vi "EOL CAN_Send_Two_Part_Message (2).vi"(0 "Write Session in":refnum<k21>, 1 "Rx Arbitration Id":u32=402522244 format="%.0x", 5 "Read Session in":refnum<k21>, 7 "Tx CAN frame 1":T1={"timestamp"=timestamp(0 s since 1904-01-01), "payload"=[2, 39, 3, 85, 85, 85, 85, 85], "identifier"=402391172, "type"=0, "extended?"=TRUE, "echo?"=FALSE} {"payload" format="%x"; "timestamp" format="%<%.7X\n%x>T"; "type" items=["CAN Data"=0, "CAN Remote"=1, "CAN Bus Error"=2, "CAN 2.0 Data"=8, "CAN FD Data"=16, "CAN FD+BRS Data"=24, "J1939 Data"=192, "Delay"=224, "Log Trigger"=225, "Start Trigger"=226]; "identifier" format="%x"}, 9 "Tx CAN frame 2":T1={"timestamp"=timestamp(0 s since 1904-01-01), "payload"=[2, 39, 3, 85, 85, 85, 85, 85], "identifier"=402391172, "type"=0, "extended?"=TRUE, "echo?"=FALSE} {"payload" format="%x"; "timestamp" format="%<%.7X\n%x>T"; "type" items=["CAN Data"=0, "CAN Remote"=1, "CAN Bus Error"=2, "CAN 2.0 Data"=8, "CAN FD Data"=16, "CAN FD+BRS Data"=24, "J1939 Data"=192, "Delay"=224, "Log Trigger"=225, "Start Trigger"=226]; "identifier" format="%x"}, 11 "error in (no error)":errorcluster, 12 "Retries":i32=1, 13 "Msg Wait Time":u32=100) -> (4 "Response Good?":bool, 6 "Rx Data":u8[](array[numeric]), 10 "TxRx Data":string[][](array[string]), 15 "error out":errorcluster)   [LabVIEW 2018]
uses:
  <vilib>/xnet/xnet.llb/XNET Frame CAN.ctl
  <vilib>/xnet/xnet.llb/XNET Frame Type CAN.ctl
  <vilib>/xnet/xnet.llb/XNET Write (Frame CAN).vi
  <vilib>/xnet/xnet.llb/XNET Read (Frame CAN).vi
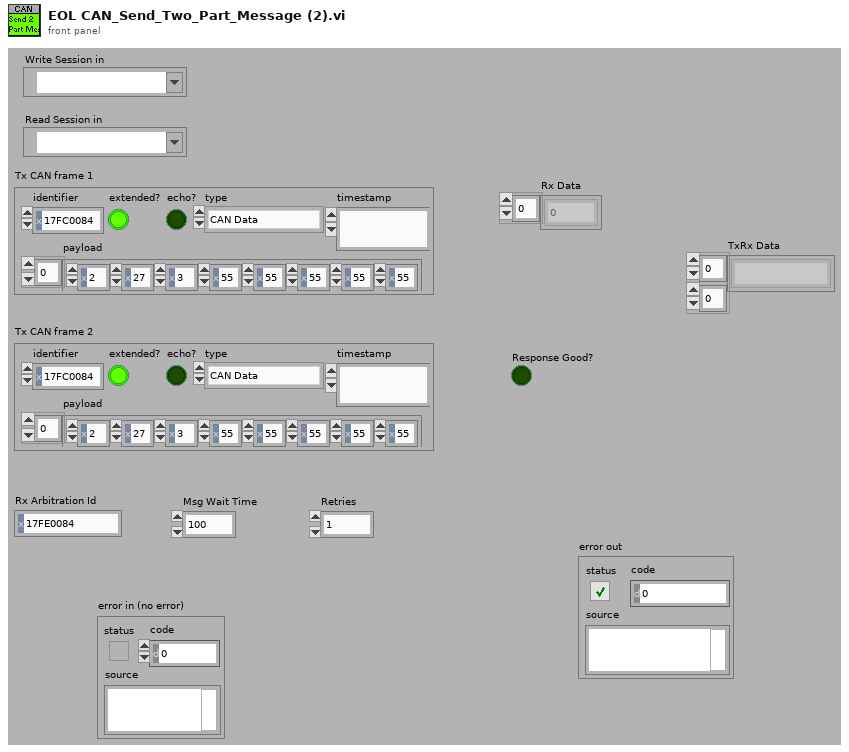
[diagram p1: front panel]
types:
  T1 = typedef "XNET Frame CAN.ctl" = cluster{"timestamp":timestamp, "payload":u8[], "identifier":u32, "type":T2, "extended?":bool, "echo?":bool}
  T2 = typedef "XNET Frame Type CAN.ctl" = u8
  T3 = cluster{"Write Session in":refnum<k21>, "Read Session in":refnum<k21>, "Tx CAN frame 1":T1, "Tx CAN frame 2":T1, "Rx Arbitration Id":u32, "Retry Counter":i32, "Rx Data":u8[], "Response Good?":bool, "TxRx Data":string[][], "Rx Bytes Length":u8, "error in (no error)":errorcluster}
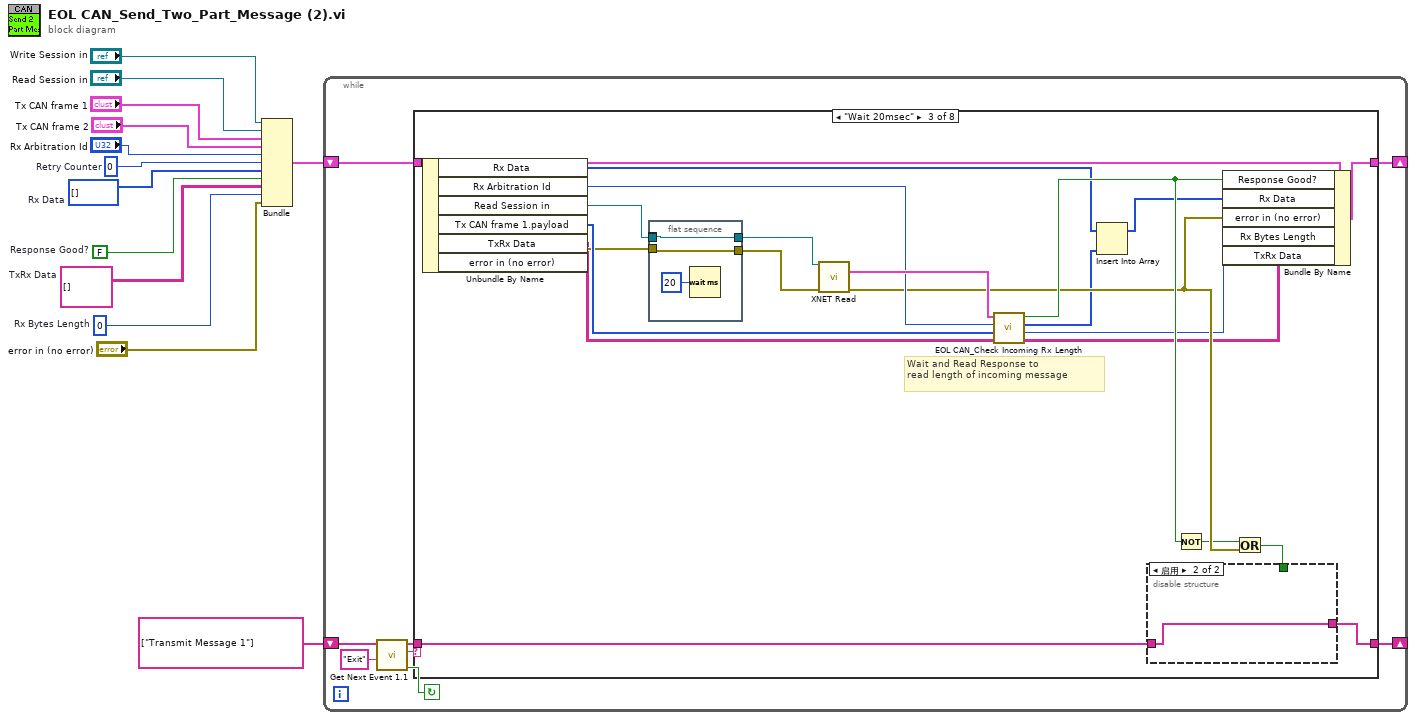
[diagram p0: block diagram]
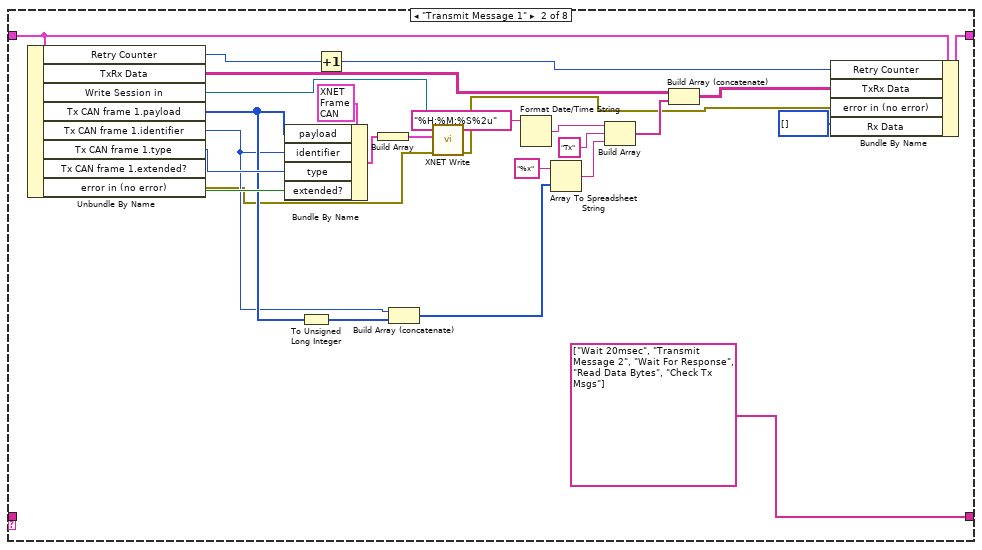
[diagram p3: hidden frame]
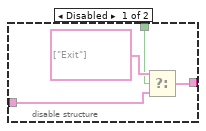
[diagram p4: hidden frame]
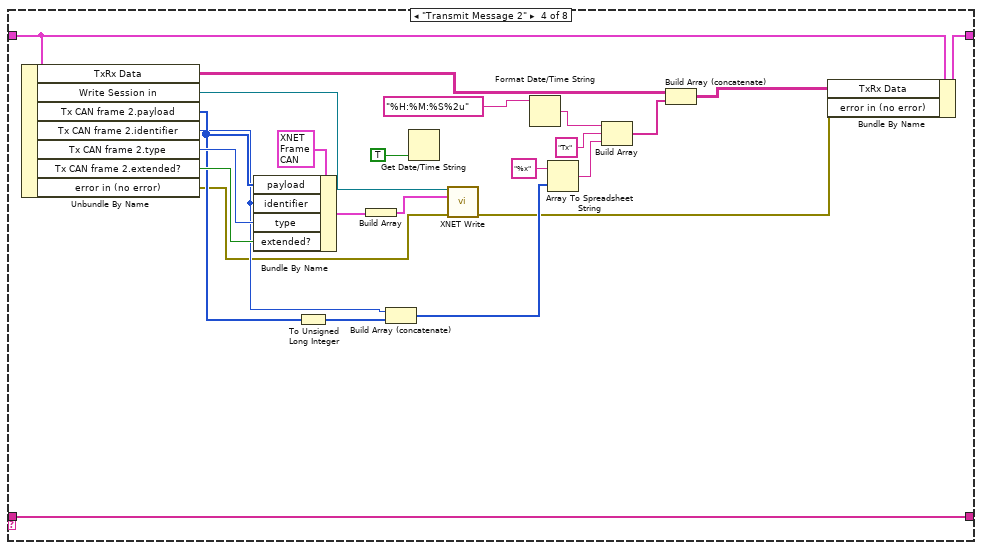
[diagram p5: hidden frame]
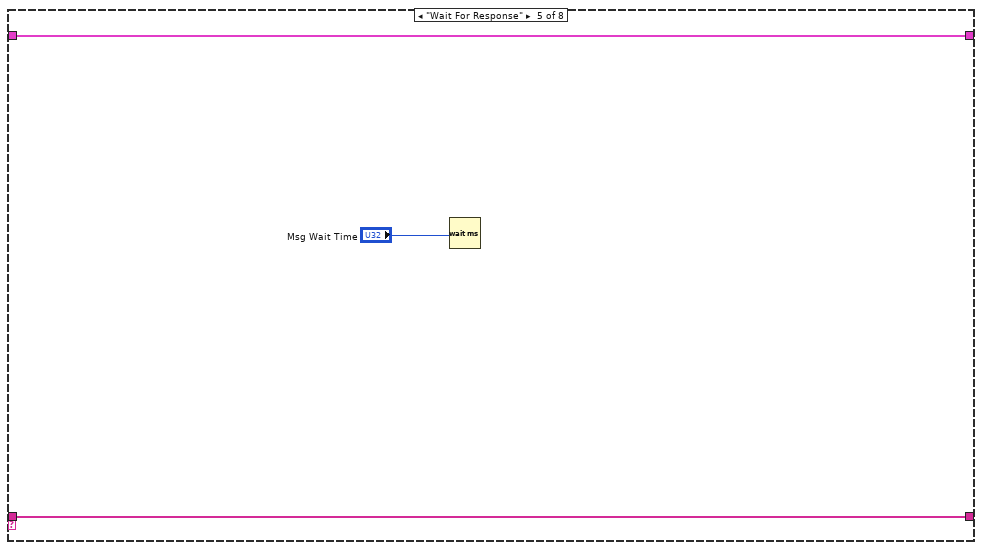
[diagram p6: hidden frame]
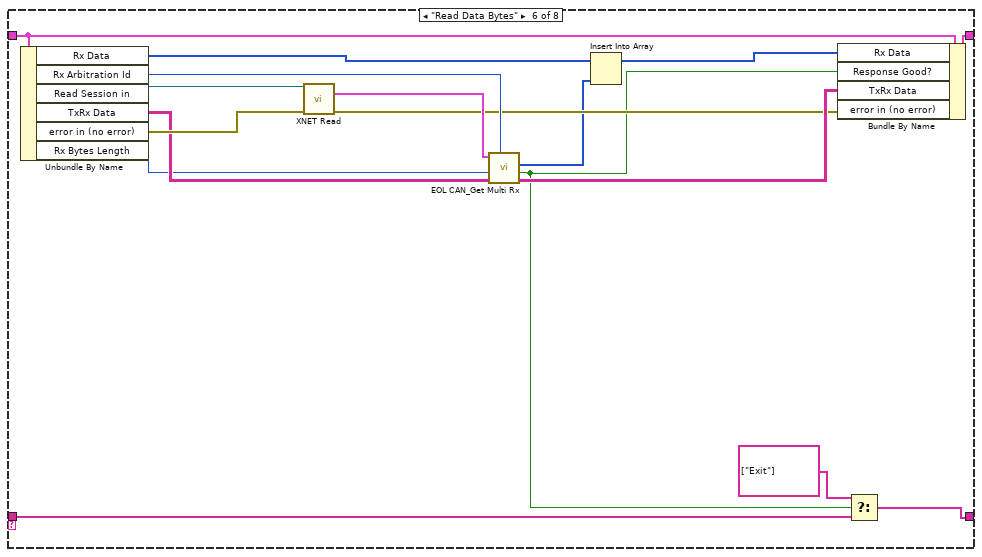
[diagram p7: hidden frame]
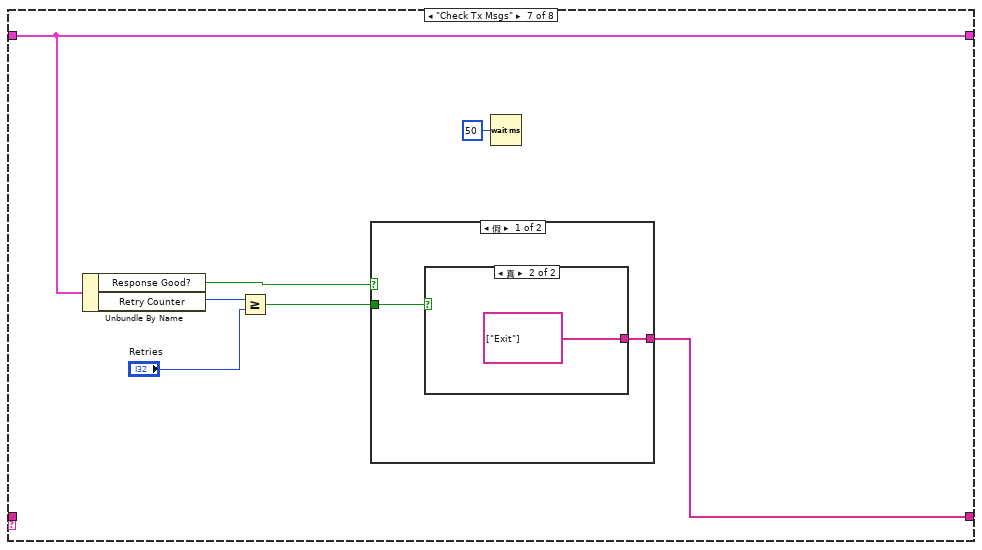
[diagram p8: hidden frame]
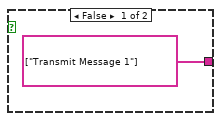
[diagram p9: hidden frame]
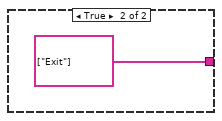
[diagram p10: hidden frame]
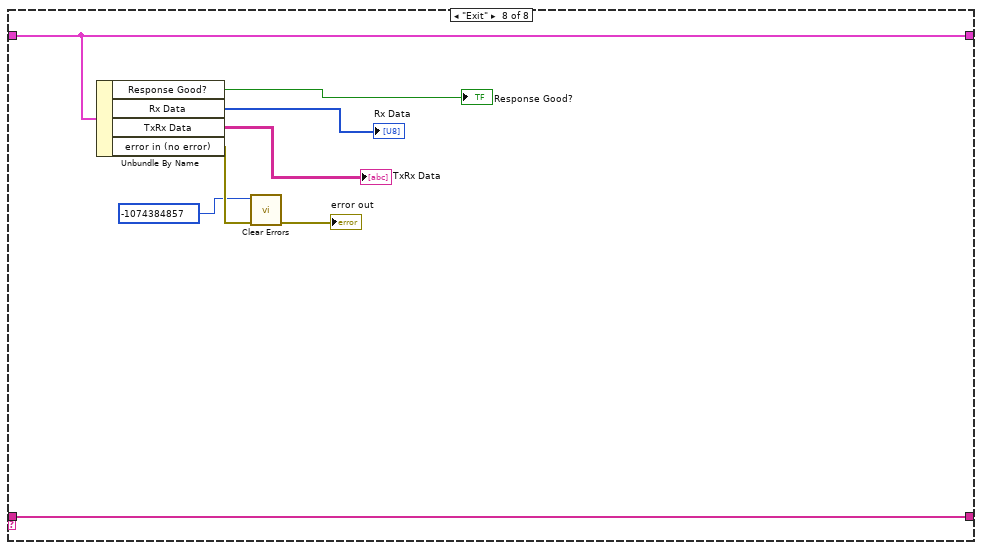
[diagram p11: hidden frame]
diagram:
  w1 = u8[] []  # Rx Data
  w2 = u8 0  # Rx Bytes Length
  w9 = string[][] []  # TxRx Data
  w10 = FALSE  # Response Good?
  w12 = 0  # Retry Counter
  n1 = Bundle("Write Session in"="Write Session in", "Read Session in"="Read Session in", "Tx CAN frame 1"="Tx CAN frame 1", "Tx CAN frame 2"="Tx CAN frame 2", "Rx Arbitration Id"="Rx Arbitration Id", "Retry Counter"=w12, "Rx Data"=w1, "Response Good?"=w10, "TxRx Data"=w9, "Rx Bytes Length"=w2, "error in (no error)"="error in (no error)") -> (w11:T3)  [unwired: 1 in]
  n2 = while {
    shift-right: [w18] -> _
    shift-left: string[] ["Transmit Message 1"] ("event queue out") -> [w17]
    shift-right: [w15] -> _
    shift-left: w11 -> [w16]
    stop <- w21 continue-if-true
    n3 = call "Get Next Event 1.1.vi"("Exit Event"="Exit", "event queue in"=w17) -> ("Condition (Exit:F)"=w21:bool, "next event"=w20:string, "event queue out"=w19:string[])  [unwired: 6 in, 1 out]
    n4 = case shown="\"Wait 20msec\"" w20 {
      tunnel: w19 -> [w23 _ w63 w102 w104 w112 _ w142]
      tunnel: [w23 string[] ["Wait 20msec", "Transmit Message 2", "Wait For Response", "Read Data Bytes", "Check Tx Msgs"] ("event queue out") w62 w102 w104 w111 w127 w142] -> w18
      tunnel: w16 -> [w22 w47 w65 w92 w105 w122 w125 w141]
      tunnel: [w22 w45 w64 w91 w105 w121 w125 w141] -> w15
      frame "Error", Default {
      }
      frame "Transmit Message 1" {
        n5 = Unbundle By Name(w47) -> ("Retry Counter"=w48:i32, "TxRx Data"=w38:string[][], "Write Session in"=w27:refnum<k21>, "Tx CAN frame 1.payload"=w31:u8[], "Tx CAN frame 1.identifier"=w30:u32, "Tx CAN frame 1.type"=w33:T2, "Tx CAN frame 1.extended?"=w32:bool, "error in (no error)"=w29:errorcluster)
        n6 = Bundle By Name(cluster=T1 {"timestamp"=timestamp(0 s since 1904-01-01), "payload"=[], "identifier"=0, "type"=0, "extended?"=FALSE, "echo?"=FALSE} ("CAN frame"), "payload"=w31, "identifier"=w30, "type"=w33, "extended?"=w32) -> (w34:T1)
        n7 = To Unsigned Long Integer(number=w31) -> (unsigned 32bit integer=w44:u32[])
        n8 = Increment(x=w48) -> (x+1=w46:i32)
        n9 = Build Array(w34) -> (w35:T1[])
        n10 = Build Array (concatenate)(w30, w44) -> (w39:u32[])
        n11 = call-poly <vilib>:"XNET Write.vi"("session in"=w27, "data"=w35, "error in (no error)"=w29) -> ("error out"=w28:errorcluster)  [unwired: 11 in, 1 out]
        n12 = Format Date/Time String(time format string (%c)="%H:%M:%S%2u" ("时间格式字符串(%c)")) -> (date/time string=w24:string)  [unwired: 2 in]
        n13 = Array To Spreadsheet String(array=w39, 3:"%x" ("format string")) -> (spreadsheet string=w42:string)  [unwired: 1 in]
        n14 = Build Array(w24, "Tx" ("format string"), w42) -> (w43:string[])
        n15 = Build Array (concatenate)(w38, w43) -> (w37:string[][])
        n16 = Bundle By Name(cluster=w47, "Retry Counter"=w46, "TxRx Data"=w37, "error in (no error)"=w28, "Rx Data"=u8[] []) -> (w45:T3)
      }
      frame "Wait 20msec" {
        # "Wait and Read Response to\nread length of incoming message"
        n17 = Unbundle By Name(w65) -> ("Rx Data"=w54:u8[], "Rx Arbitration Id"=w68:u32, "Read Session in"=w51:refnum<k21>, "Tx CAN frame 1.payload"=w70:u8[], "TxRx Data"=w57:string[][], "error in (no error)"=w61:errorcluster)
        n18 = flat-sequence {
          tunnel: w61 -> [w77]
          tunnel: [w77] -> w60
          tunnel: [w76] -> _
          tunnel: w51 -> [w76]
          tunnel: [w76] -> w50
          frame #0 {
            n19 = Wait (ms)(milliseconds to wait=u32 20) -> ()  [unwired: 1 out]
          }
        }
        n20 = call-poly <vilib>:"XNET Read.vi"("session in"=w50, "error in (no error)"=w60) -> ("data"=w69:T1[], "error out"=w59:errorcluster)  [unwired: 10 in, 2 out]
        n21 = call "EOL CAN_Check Incoming Rx Length.vi"("TxRx Data in"=w57, "Tx"=w70, "Rx Arbitration Id"=w68, "data"=w69) -> ("TxRx Data out"=w55:string[][], "Rx Bytes"=w56:u8, "Rx Data"=w53:u8[], "Response Good?"=w67:bool)  [unwired: 4 in]
        n22 = Insert Into Array(array=w54, new element=w53) -> (w52:u8[])  [unwired: 1 in]
        n23 = Not(x=w67) -> (.not. x?=w58:bool)
        n24 = Bundle By Name(cluster=w65, "Response Good?"=w67, "Rx Data"=w52, "error in (no error)"=w59, "Rx Bytes Length"=w56, "TxRx Data"=w55) -> (w64:T3)
        n25 = Or(x=w58, y=w59) -> (x .or. y?=w66:bool)
        n26 = disable-structure shown="启用" {
          disable-tunnel: w66 -> [w73 _]
          disable-tunnel: w63 -> [w72 w75]
          disable-tunnel: [w71 w75] -> w62
          frame Disabled {
            n27 = Select(t=string[] ["Exit"], s=w73, f=w72) -> (s? t:f=w71:string[])
          }
          frame Enabled {
          }
        }
      }
      frame "Transmit Message 2" {
        n28 = Unbundle By Name(w92) -> ("TxRx Data"=w94:string[][], "Write Session in"=w90:refnum<k21>, "Tx CAN frame 2.payload"=w85:u8[], "Tx CAN frame 2.identifier"=w84:u32, "Tx CAN frame 2.type"=w87:T2, "Tx CAN frame 2.extended?"=w86:bool, "error in (no error)"=w82:errorcluster)
        n29 = Bundle By Name(cluster=T1 {"timestamp"=timestamp(0 s since 1904-01-01), "payload"=[], "identifier"=0, "type"=0, "extended?"=FALSE, "echo?"=FALSE} ("CAN frame"), "payload"=w85, "identifier"=w84, "type"=w87, "extended?"=w86) -> (w89:T1)
        n30 = To Unsigned Long Integer(number=w85) -> (unsigned 32bit integer=w101:u32[])
        n31 = Build Array(w89) -> (w83:T1[])
        n32 = Build Array (concatenate)(w84, w101) -> (w95:u32[])
        n33 = Get Date/Time String(want seconds? (F)=TRUE) -> ()  [unwired: 2 in, 2 out]
        n34 = call-poly <vilib>:"XNET Write.vi"("session in"=w90, "data"=w83, "error in (no error)"=w82) -> ("error out"=w81:errorcluster)  [unwired: 11 in, 1 out]
        n35 = Format Date/Time String(time format string (%c)="%H:%M:%S%2u" ("时间格式字符串(%c)")) -> (date/time string=w80:string)  [unwired: 2 in]
        n36 = Array To Spreadsheet String(array=w95, 3:"%x" ("format string")) -> (spreadsheet string=w99:string)  [unwired: 1 in]
        n37 = Build Array(w80, "Tx" ("format string"), w99) -> (w100:string[])
        n38 = Build Array (concatenate)(w94, w100) -> (w93:string[][])
        n39 = Bundle By Name(cluster=w92, "TxRx Data"=w93, "error in (no error)"=w81) -> (w91:T3)
      }
      frame "Wait For Response" {
        n40 = Wait (ms)(milliseconds to wait="Msg Wait Time") -> ()  [unwired: 1 out]
      }
      frame "Read Data Bytes" {
        n41 = Unbundle By Name(w122) -> ("Rx Data"=w109:u8[], "Rx Arbitration Id"=w117:u32, "Read Session in"=w120:refnum<k21>, "TxRx Data"=w115:string[][], "error in (no error)"=w118:errorcluster, "Rx Bytes Length"=w114:u8)
        n42 = call-poly <vilib>:"XNET Read.vi"("session in"=w120, "error in (no error)"=w118) -> ("data"=w119:T1[], "error out"=w110:errorcluster)  [unwired: 10 in, 2 out]
        n43 = call "EOL CAN_Get Multi Rx.vi"("Rx Arbitration Id"=w117, "TxRx Data in"=w115, "Rx Bytes Length"=w114, "data"=w119) -> ("TxRx Data out"=w116:string[][], "Response Good?"=w106:bool, "Rx Data"=w108:u8[])  [unwired: 5 in]
        n44 = Insert Into Array(array=w109, new element=w108) -> (w107:u8[])  [unwired: 1 in]
        n45 = Bundle By Name(cluster=w122, "Rx Data"=w107, "Response Good?"=w106, "TxRx Data"=w116, "error in (no error)"=w110) -> (w121:T3)
        n46 = Select(t=string[] ["Exit"], s=w106, f=w112) -> (s? t:f=w111:string[])
      }
      frame "Check Tx Msgs" {
        n47 = Unbundle By Name(w125) -> ("Response Good?"=w128:bool, "Retry Counter"=w129:i32)
        n48 = Greater Or Equal?(x=w129, y="Retries") -> (x >= y?=w126:bool)
        n49 = case shown="假" w128 {
          tunnel: [w130 string[] ["Exit"] ("event queue out")] -> w127
          tunnel: w126 -> [w131 _]
          frame False {
            n50 = case shown="真" w131 {
              tunnel: [string[] ["Transmit Message 1"] ("f") string[] ["Exit"] ("event queue out")] -> w130
              frame False {
              }
              frame True {
              }
            }
          }
          frame True {
          }
        }
        n51 = Wait (ms)(milliseconds to wait=u32 50) -> ()  [unwired: 1 out]
      }
      frame "Exit" {
        n52 = Unbundle By Name(w141) -> ("Response Good?"=→"Response Good?":bool, "Rx Data"=→"Rx Data":u8[], "TxRx Data"=→"TxRx Data":string[][], "error in (no error)"=w138:errorcluster)
        n53 = call <vilib>:"Clear Errors.vi"("error in (no error)"=w138, "specific error code to clear (0: all)"=-1074384857) -> ("error out"=→"error out":errorcluster)  [unwired: 4 in, 1 out]
      }
    }
  }
